vi "Expt 9.vi"() -> ()   [LabVIEW 2020]
uses:
  <vilib>/numeric/Random Number (Range) U64.vi
  <vilib>/numeric/sub_Random U32.vi
panel:
  out "Waveform Graph":u64[](graph)
  in  "Number of samples":i32
  out "Waveform Chart":u64(graph)
  out "current time":timestamp
  out "x^2 3":dbl
  in  "x 3":dbl
  in  "y 3":dbl
  out "x+y 3":dbl
  out "x^2":dbl
  out "x+y":dbl
  in  "y":dbl
  in  "x":dbl
  # "1)"
  # "Flat sequence"
  # "Stacked Sequence"
  # "2)"
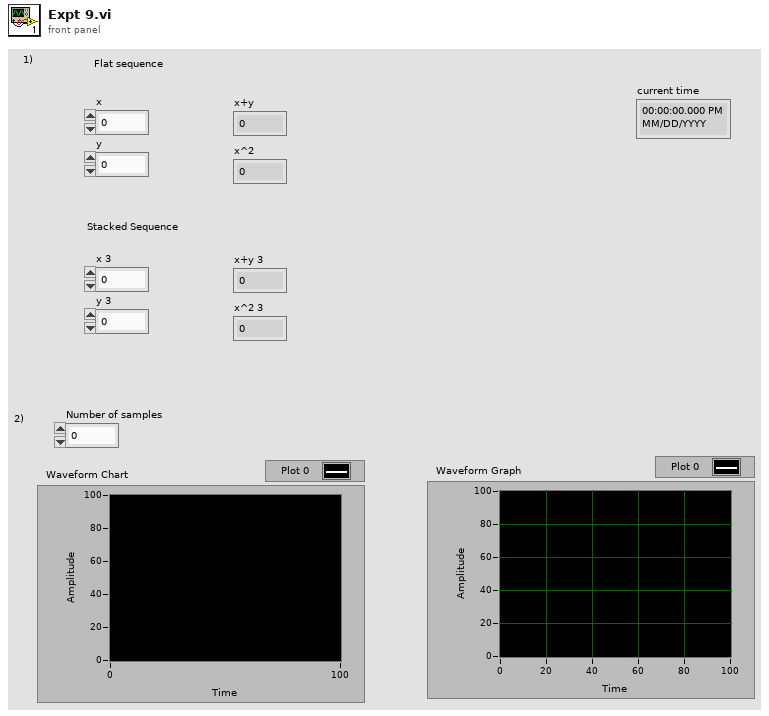
[diagram p1: front panel]
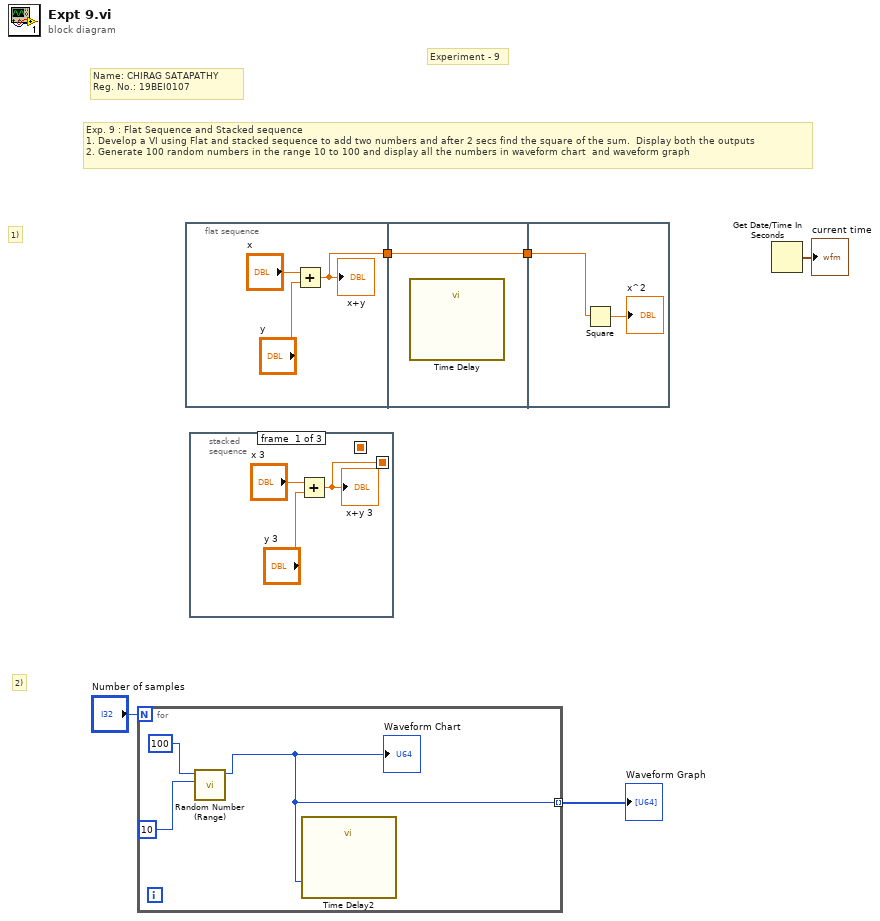
[diagram p0: block diagram]
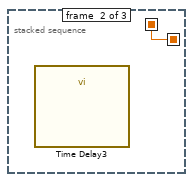
[diagram p2: hidden frame]
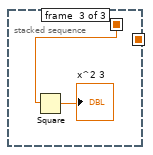
[diagram p3: hidden frame]
diagram:
  # "2)"
  # "1)"
  # "Name: CHIRAG SATAPATHY\nReg. No.: 19BEI0107"
  # "Experiment - 9"
  # "Exp. 9 : Flat Sequence and Stacked sequence\n1. Develop a VI using Flat and stacked sequence to add two numbers and after 2 secs find the square of the sum.  Display both the outputs\n2. Generate 100 random numbers in the range 10 to 100 and display all the numbers in waveform chart  and waveform graph"
  n1 = for {
    N: "Number of samples" -> [_]
    tunnel: [w6] -> w1 mode=indexing
    n2 = call-poly <vilib>:"Random Number (Range).vi"("lower bound (0)"=u64 10, "upper bound (100)"=u64 100) -> ("number"=w6:u64)  [unwired: 9 in]
    "Waveform Chart" <- w6
    n3 = call "Time Delay2"("Delay Time (s)"=w6) -> ()  [unwired: 10 in, 1 out]
  }
  "Waveform Graph" <- w1
  n4 = flat-sequence {
    tunnel: [w9] -> w5
    tunnel: w5 -> [w12]
    tunnel: [w12] -> w4
    tunnel: w4 -> [w14]
    frame #0 {
      n5 = Add(x="x", y="y") -> (x+y=w9:dbl)
      "x+y" <- w9
    }
    frame #1 {
      n6 = call "Time Delay"() -> ()  [unwired: 11 in, 1 out]
    }
    frame #2 {
      n7 = Square(x=w14) -> (x^2=→"x^2":dbl)
    }
  }
  n8 = stacked-sequence {
    seq-local: [w15 _ _] -> [_ w18 _]
    seq-local: [_ w18 _] -> [_ _ w20]
    frame #0 {
      n9 = Add(x="x 3", y="y 3") -> (x+y=w15:dbl)
      "x+y 3" <- w15
    }
    frame #1 {
      n10 = call "Time Delay3"() -> ()  [unwired: 11 in, 1 out]
    }
    frame #2 {
      n11 = Square(x=w20) -> (x^2=→"x^2 3":dbl)
    }
  }
  n12 = Get Date/Time In Seconds() -> (seconds since 1Jan1904=→"current time":timestamp)
